vi "GenerateImmediateCommand.vi"(8 "error in":errorcluster, 11 "T560Trigger in":refnum<class "T560Trigger.lvclass">) -> (0 "error out":errorcluster, 3 "T560Trigger out":refnum<class "T560Trigger.lvclass">)   [LabVIEW 2013, in "T560Trigger.lvclass"]
uses:
  T560Trigger.lvclass
  T560Trigger.lvclass/T560Trigger.ctl
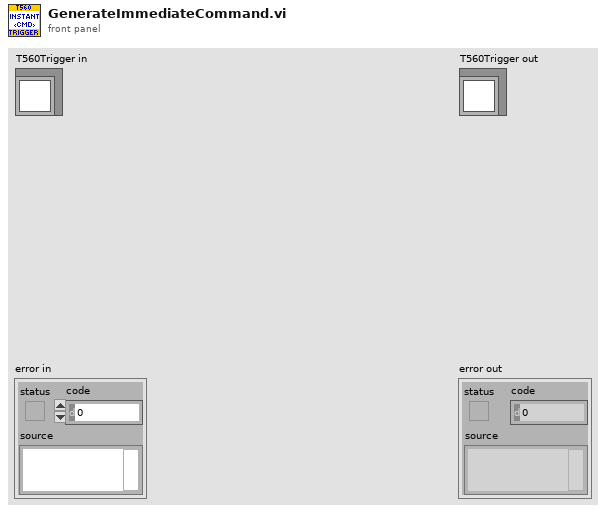
[diagram p1: front panel]
types:
  T1 = typedef "TriggerSource.ctl" = enum16{"Rising", "Falling", "Internal 80MHz", "Internal DDS", "Remote", "Disabled"}
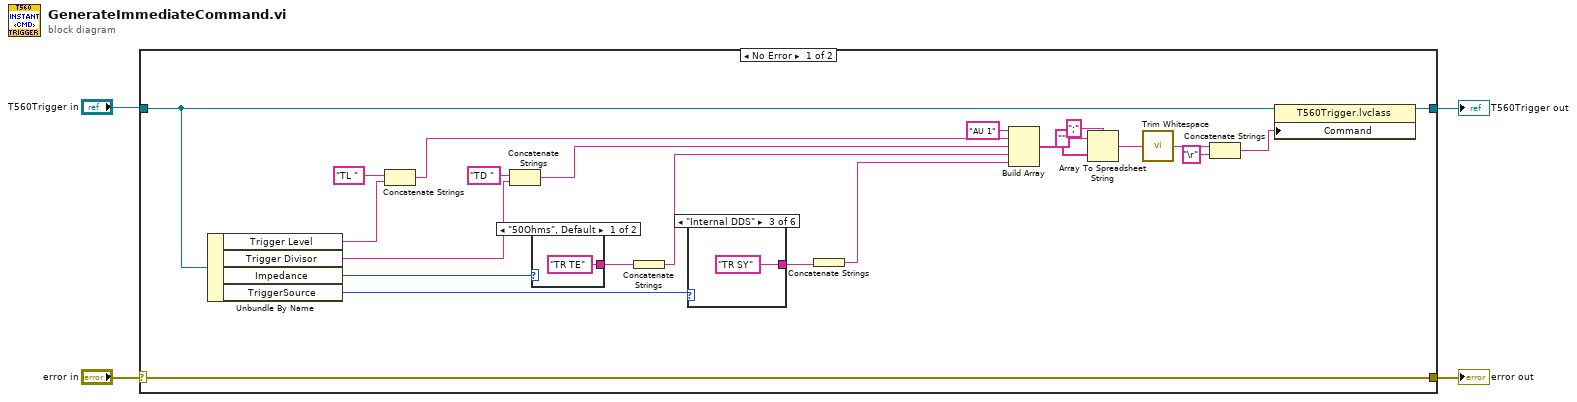
[diagram p0: block diagram]
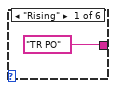
[diagram p2: hidden frame]
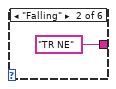
[diagram p3: hidden frame]
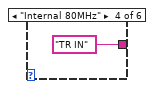
[diagram p4: hidden frame]
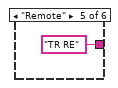
[diagram p5: hidden frame]
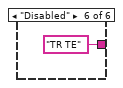
[diagram p6: hidden frame]
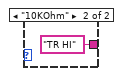
[diagram p7: hidden frame]
diagram:
  n1 = case shown="No Error" "error in" {
    selector: "error in" -> [w27 w37]
    tunnel: [w27 w37] -> w2
    tunnel: [w7 w36] -> w1
    tunnel: "T560Trigger in" -> [w19 w36]
    frame No Error {
      n2 = Unbundle By Name(w19) -> ("Trigger Level"=w18:string, "Trigger Divisor"=w17:string, "Impedance"=w16:enum16{"10KOhm", "50Ohms"}, "TriggerSource"=w6:T1)
      n3 = Concatenate Strings("TL ", w18) -> (w25:string)
      n4 = Concatenate Strings("TD ", w17) -> (w26:string)
      n5 = case shown="\"50Ohms\", Default" w16 {
        tunnel: ["TR TE" "TR HI"] -> w21
        frame "50Ohms", Default {
        }
        frame "10KOhm" {
        }
      }
      n6 = Concatenate Strings(w21) -> (w22:string)
      n7 = case shown="\"Internal DDS\"" w6 {
        tunnel: ["TR PO" "TR NE" "TR SY" "TR IN" "TR RE" "TR TE"] -> w5
        frame "Rising" {
        }
        frame "Falling" {
        }
        frame "Internal DDS" {
        }
        frame "Internal 80MHz" {
        }
        frame "Remote" {
        }
        frame "Disabled" {
        }
      }
      n8 = Concatenate Strings(w5) -> (w23:string)
      n9 = Build Array("AU 1" ("element"), w25, w26, w22, w23) -> (w14:string[])
      n10 = Array To Spreadsheet String(delimiter (Tab)=";", array=w14, 3:"" ("format string")) -> (spreadsheet string=w15:string)
      n11 = call <vilib>:"Trim Whitespace.vi"("string"=w15) -> ("trimmed string"=w11:string)  [unwired: 1 in]
      n12 = Concatenate Strings(w11, "\r" ("string")) -> (w8:string)
      n13 = property class="T560Trigger.lvclass"(reference=w19, "Command"=w8) -> (reference out=w7:refnum<class "T560Trigger.lvclass">)  [unwired: 1 in, 1 out]
    }
    frame Error {
    }
  }
  "error out" <- w2
  "T560Trigger out" <- w1
